vi "Teleop.vi"(10 "Match Info":T2={"Autonomous Elapsed Seconds"=0.0, "TeleOp Elapsed Seconds"=0.0, "Disabled Elapsed Seconds"=0.0, "Visited Autonomous"=FALSE, "Visited TeleOp"=FALSE, "Visited Disabled"=FALSE, "Autonomous Settings"={"Autonomous Style"=enum."Independent", "VI Refnum"=refnum}}, 11 "Call Context":T3) -> ()   [LabVIEW 2015]
doc: "This VI is called for each TeleOp packet received from the DS where the robot is not disabled. It is often used to read from the joysticks and update I/O or to update setpoints for timed control loops. It should complete and return within 20 milliseconds or it may miss DS packets."
uses:
  <vilib>/Rock Robotics/WPI/DriverStation/WPI_DriverStationDerivedRobotMode.ctl
  <vilib>/Rock Robotics/WPI/DriverStation/WPI_DriverStationMatch Info.ctl
  <vilib>/Rock Robotics/WPI/CAN/TalonSRX/WPI_CANTalonSRX_BrakeOverride.ctl
  <vilib>/Rock Robotics/WPI/CAN/TalonSRX/WPI_CANTalonSRX_APIControlMode.ctl
  <vilib>/Rock Robotics/WPI/Utilities/WPI_GetSetVariantRefNum.vi
  <vilib>/Rock Robotics/Network Tables/SD Write Number.vi
  <vilib>/Rock Robotics/Network Tables/NT Write Number.vi
  <vilib>/Rock Robotics/Network Tables/SD Write Boolean.vi
  <vilib>/Rock Robotics/WPI/Solenoid/Deprecated/WPI_SolenoidSetBool.vi
  Robot Global Data.vi
  <vilib>/addons/control/pid/pid.llb/PID (DBL).vi
  navX Library v2/navX Library v2.lvlib
  <vilib>/addons/control/pid/NI_PID_pid.lvlib
panel:
  in  "RPM":dbl
  in  "Aiming Gains":T1={"proportional gain (Kc)"=1.0, "integral time (Ti, min)"=0.01, "derivative time (Td, min)"=0.0} {"derivative time (Td, min)" format="%.3f"; "integral time (Ti, min)" format="%.3f"; "proportional gain (Kc)" format="%.3f"}
  out "Displacement X":dbl
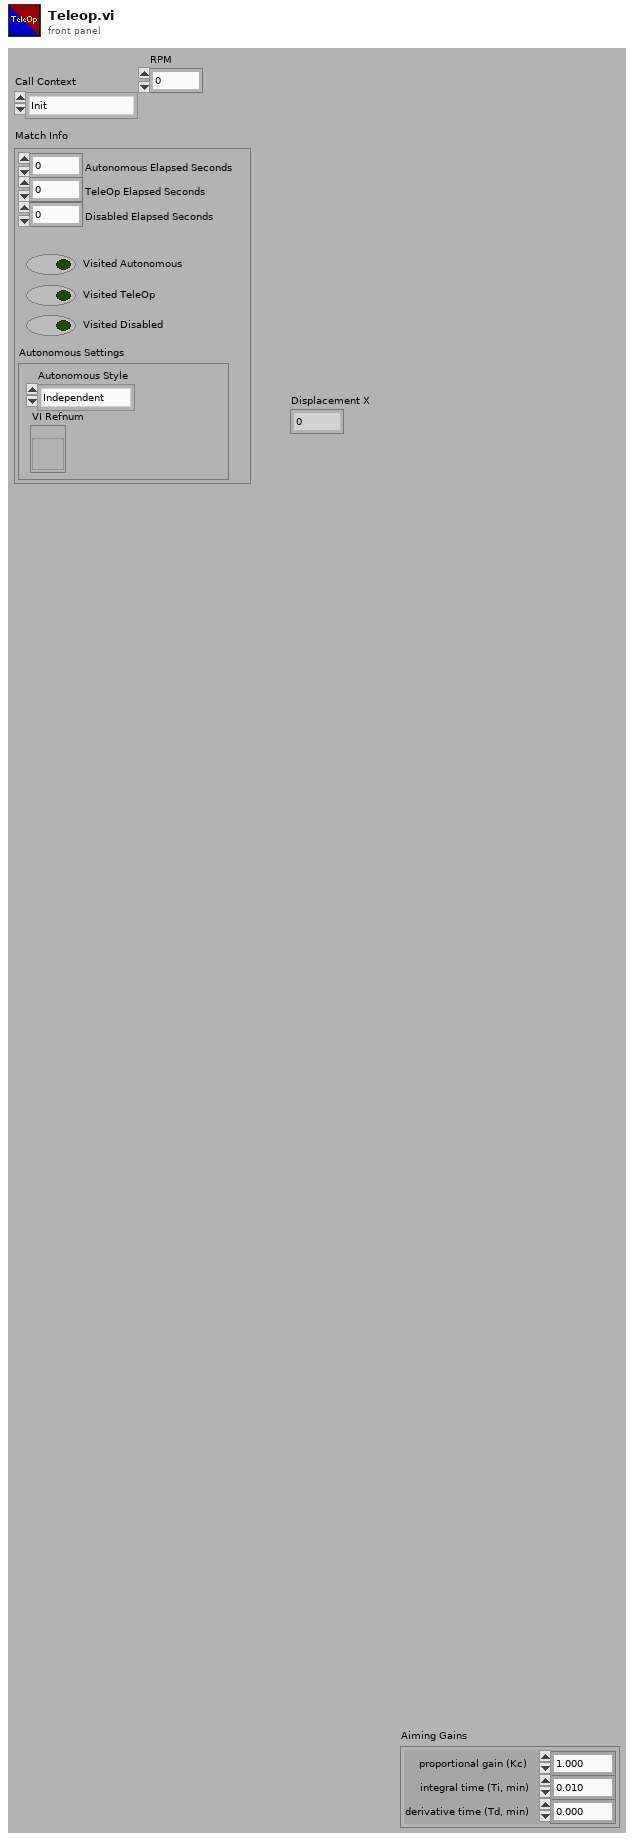
[diagram p1: front panel]
types:
  T1 = cluster{"proportional gain (Kc)":dbl, "integral time (Ti, min)":dbl, "derivative time (Td, min)":dbl}
  T2 = typedef "WPI_DriverStationMatch Info.ctl" = cluster{"Autonomous Elapsed Seconds":dbl, "TeleOp Elapsed Seconds":dbl, "Disabled Elapsed Seconds":dbl, "Visited Autonomous":bool, "Visited TeleOp":bool, "Visited Disabled":bool, "Autonomous Settings":cluster{"Autonomous Style":enum16{"Iterative", "Independent"}, "VI Refnum":refnum<vi>}}
  T3 = typedef "WPI_DriverStationDerivedRobotMode.ctl" = enum16{"Init", "Execute", "Stop"}
  T4 = typedef "WPI_CANTalonSRX_BrakeOverride.ctl" = enum8{"No Override", "Override to Coast", "Override to Brake"}
  T5 = typedef "WPI_MotorControlDeviceRef.ctl" = cluster{"DeviceStatus":errorcluster, "Type":T6, "PWM":cluster{"PWM Channel":T7, "DeadBand":T8}, "CAN":cluster{"Device Number":u8, "Control Mode":T9, "Semaphore":T10, "Max Vout":dbl, "TalonSRX Control Mode":T11}, "Invert":bool}
  T6 = typedef "WPI_MotorControlType.ctl" = enum16{"PWM", "CAN", "CANTalonSRX"}
  T7 = typedef "FPGA_DIOPWMChannel.ctl" = enum8{"PWM 0", "PWM 1", "PWM 2", "PWM 3", "PWM 4", "PWM 5", "PWM 6", "PWM 7", "PWM 8", "PWM 9", "PWM MXP 0", "PWM MXP 1", "PWM MXP 2", "PWM MXP 3", "PWM MXP 4", "PWM MXP 5", "PWM MXP 6", "PWM MXP 7", "PWM MXP 8", "PWM MXP 9", "Invalid"}
  T8 = typedef "WPI_PWMDeadband.ctl" = cluster{"Name":string, "maxPositivePwm":i32, "minPositivePwm":i32, "centerPwm":i32, "maxNegativePwm":i32, "minNegativePwm":i32, "angularRange":u16}
  T9 = typedef "WPI_CANJaguar_ControlMode.ctl" = enum8{"Percent VBus", "Current", "Speed", "Position", "Voltage"}
  T10 = typedef "Semaphore RefNum" = refnum<k1>
  T11 = typedef "WPI_CANTalonSRX_APIControlMode.ctl" = enum8{"Percent VBus", "Speed", "Position", "Slave", "Unchanged / Invalid", "Voltage Compensation", "Current", "Motion Profile"}
  T12 = typedef "navX Library v2.lvlib/Z900_navX_DeviceTypeDef.ctl" = cluster{"Interface":cluster{"Protocol":T13, "Update Rate (4Hz-60Hz)":u8, "navX Open TypeDef":variant}, "Notify Packet":refnum<notifier>, "Loop VI Refnum":refnum<vi>, "Ready to Close Occurrence Refnum":refnum<k4>}
  T13 = typedef "navX Library v2.lvlib/Z900_navX_ProtocolTypeDef.ctl" = enum16{"SERIAL", "I2C", "SPI"}
  T14 = cluster{"Yaw":dbl, "Roll":dbl, "Pitch":dbl, "Heading":dbl, "Fused Heading":dbl}
  T15 = cluster{"LinearAcceleration X":dbl, "LinearAcceleration Y":dbl, "LinearAcceleration Z":dbl}
  T16 = typedef "WPI_JoystickDevRef.ctl" = cluster{"Device":T17}
  T17 = typedef "WPI_JoystickDeviceEnum.ctl" = enum16{"USB 0", "USB 1", "USB 2", "USB 3", "USB 4", "USB 5"}
  T18 = cluster{"Velocity X":dbl, "Velocity Y":dbl, "Velocity Z":dbl, "Displacement X":dbl, "Displacement Y":dbl, "Displacement Z":dbl}
  T19 = cluster{"Axes[0]":dbl, "Axes[1]":dbl, "Axes[2]":dbl, "Axes[3]":dbl, "Axes[4]":dbl, "Axes[5]":dbl, "Axes[6]":dbl, "Axes[7]":dbl, "Axes[8]":dbl}
  T20 = cluster{"Buttons[0]":bool, "Buttons[1]":bool, "Buttons[2]":bool, "Buttons[3]":bool, "Buttons[4]":bool, "Buttons[5]":bool, "Buttons[6]":bool, "Buttons[7]":bool, "Buttons[8]":bool}
  T21 = typedef "WPI_CANTalonSRX_GlobalStatus.ctl" = cluster{"Applied Throttle":dbl, "Module Enabled":bool, "CAN Error":errorcluster, "Closed Loop Error":dbl, "Forward Limit Switch Closed":bool, "Reverse Limit Switch Closed":bool, "Sensor Position":dbl, "Sensor Velocity":dbl, "Current":dbl, "Sticky Fault - Over Temp":bool, "Sticky Fault - Under Voltage":bool, "Sticky Fault - Forward Limit":bool, "Sticky Fault - Reverse Limit":bool, "Sticky Fault - Forward Soft Limit":bool, "Sticky Fault - Reverse Soft Limit":bool, "Brake is Enabled":bool, "Encoder Position":dbl, "Encoder Velocity":dbl, "Encoder Index Count":dbl, "Encoder A Pin State":bool, "Encoder B Pin State":bool, "Encoder Index Pin State":bool, "Analog In":dbl, "Analog In Velocity":dbl, "Temperature (C)":dbl, "Battery Voltage":dbl, "Control 5 Is Supported":bool, "Current Profile Slot Select":dbl, "Pos Div 8":bool, "Vel Div 4":bool, "Pulse Width Position":i32, "Pulse Width Velocity":i32, "Pulse Width Rise To Rise (us)":i32, "Pulse Width Rise To Fall (us)":i32, "Mot Prof Active Is Under Run":bool, "Mot Prof Active Has Under Run":bool, "Mot Prof Active Is Last":bool, "Mot Prof Active Velocity Only":bool, "Mot Prof Active Is Valid":bool, "Mot Prof Buffer Is Full":bool, "Mot Prof Active Profile Slot Select":i32, "Mot Prof NextID":i32, "Mot Prof Count":i32, "Mot Prof Active Velocity":dbl, "Mot Prof Active Position":dbl, "Mot Prof Output Enable":i32}
  T22 = typedef "WPI_SolenoidDevRef.ctl" = cluster{"DevStatus":errorcluster, "Pneumatics Control Module":u8, "Forward Solenoid Channel":T23, "Reverse Solenoid Channel":T23}
  T23 = typedef "WPI_SolenoidChannel.ctl" = enum8{"Solenoid 0", "Solenoid 1", "Solenoid 2", "Solenoid 3", "Solenoid 4", "Solenoid 5", "Solenoid 6", "Solenoid 7", "Invalid"}
  T24 = typedef "WPI_RobotDriveDevRef.ctl" = cluster{"DevStatus":errorcluster, "Motors[]":T5[], "Square Inputs":bool, "Max Output":dbl}
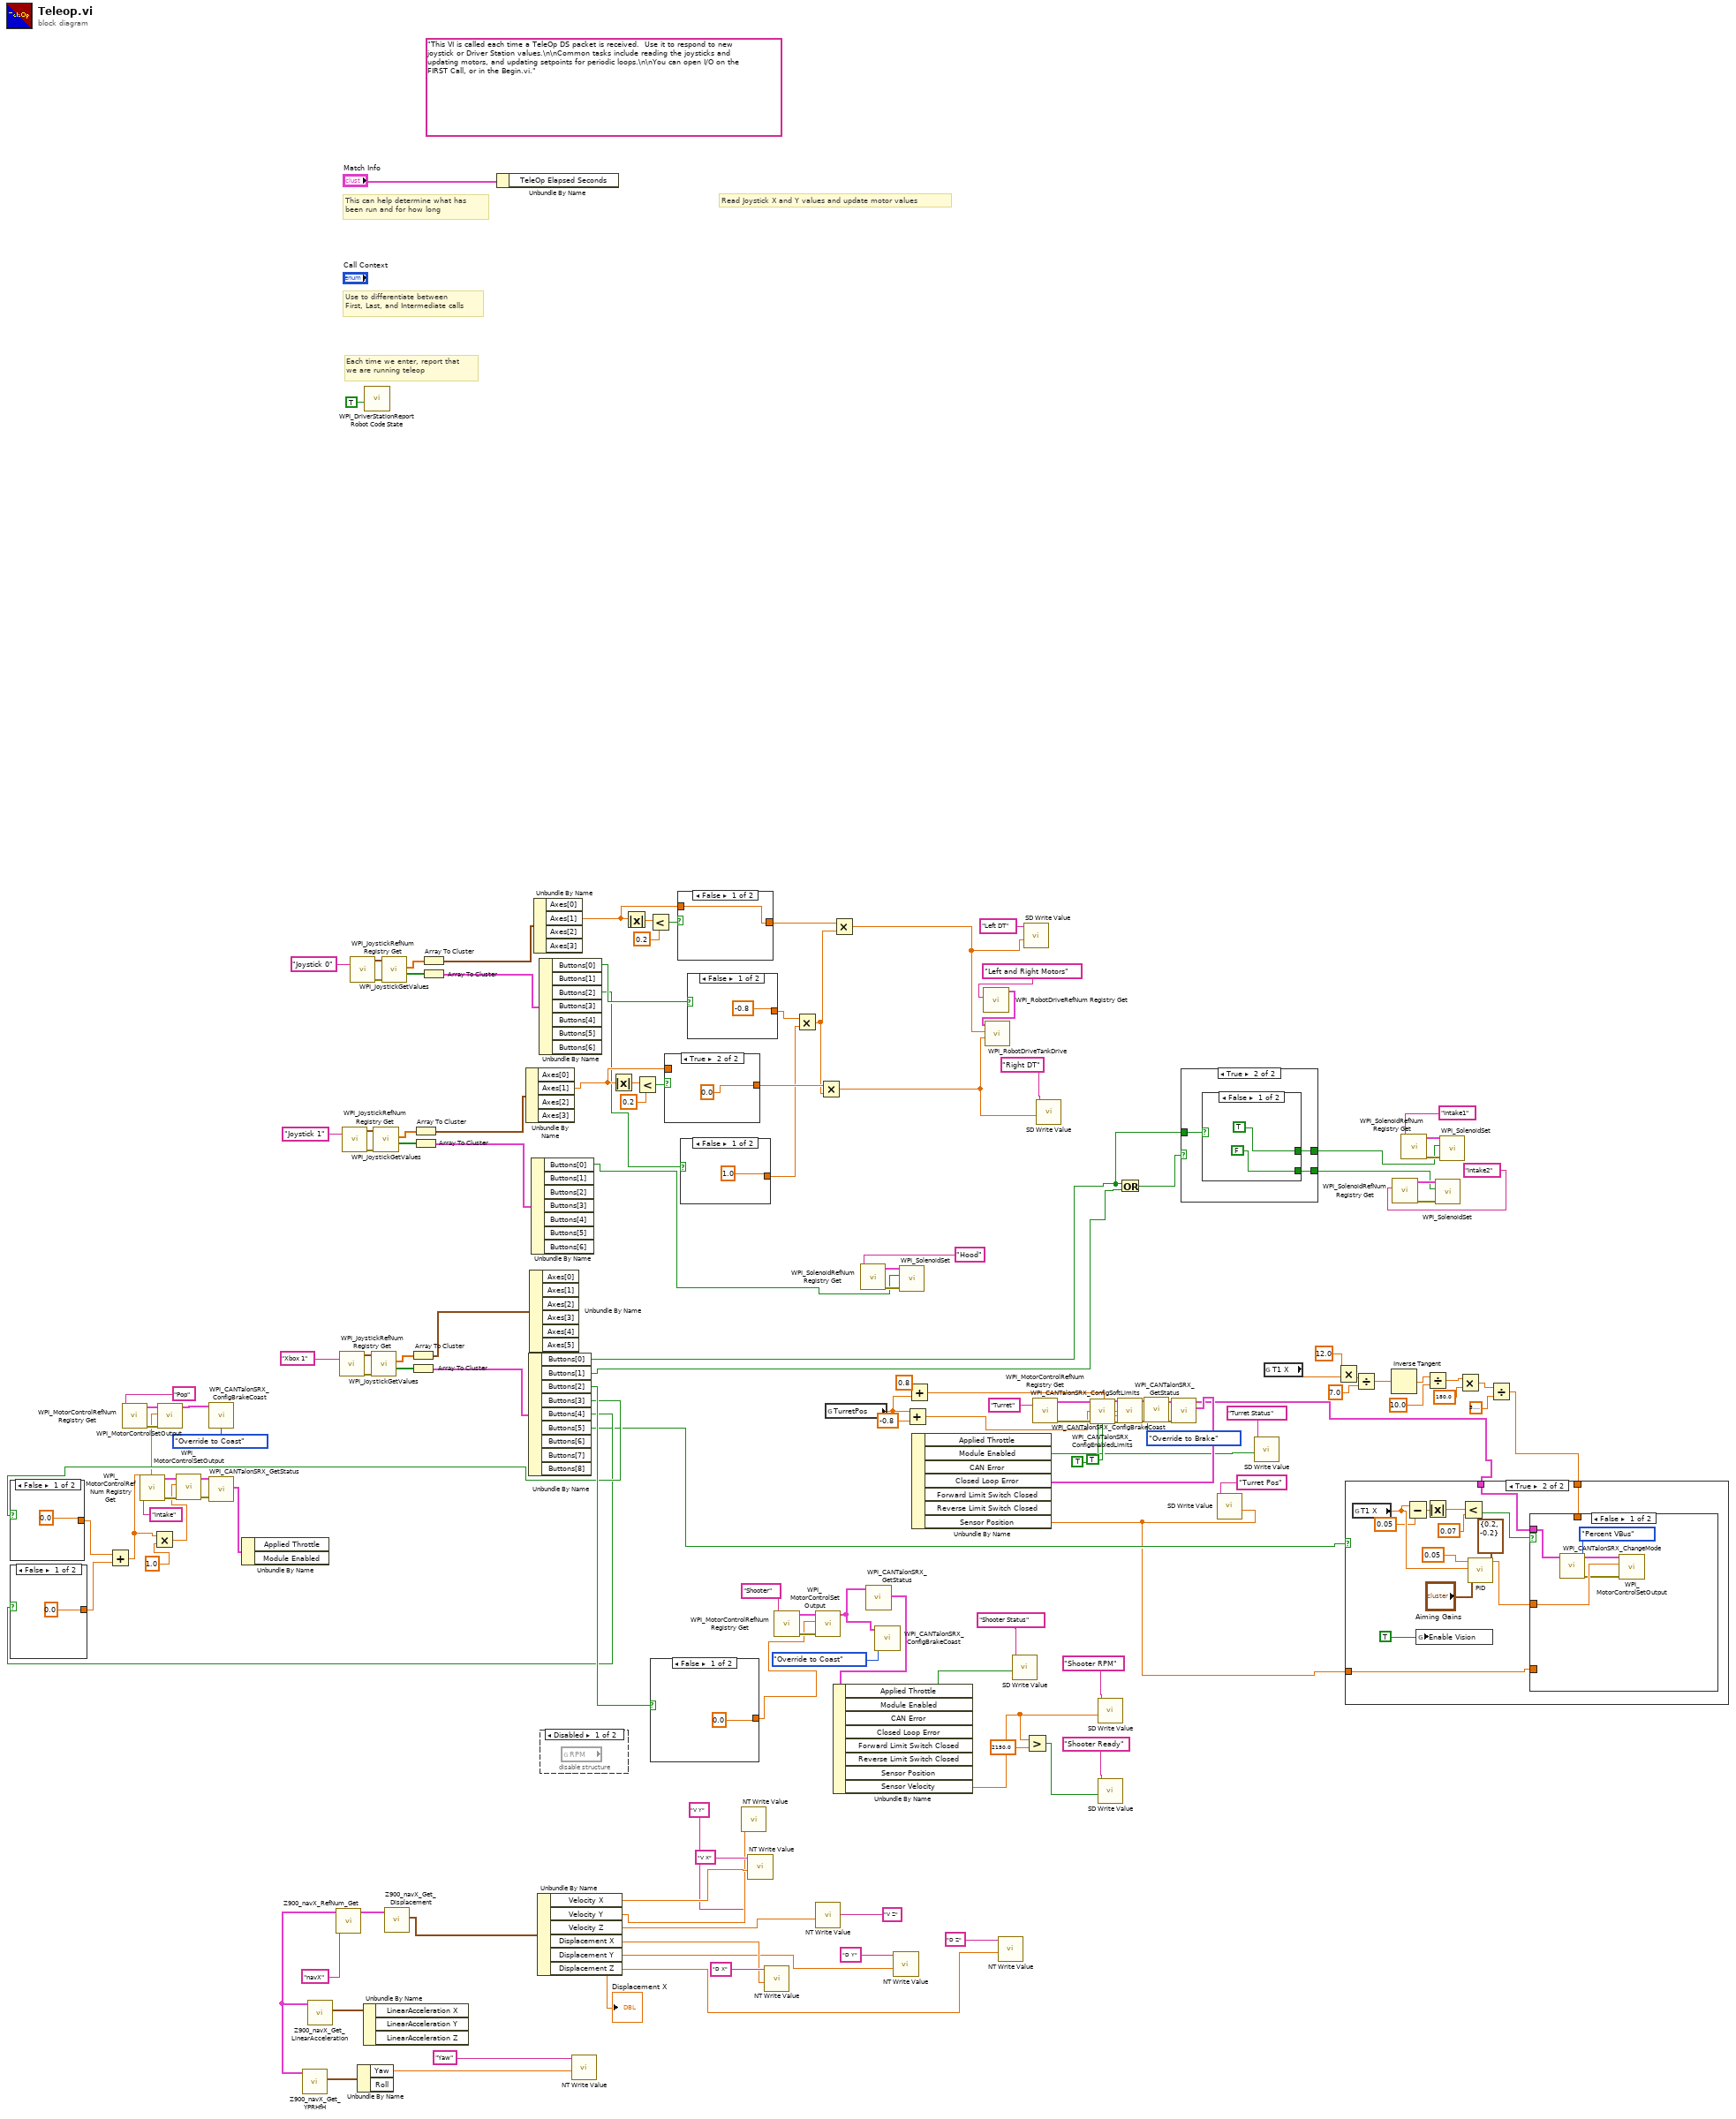
[diagram p0: block diagram]
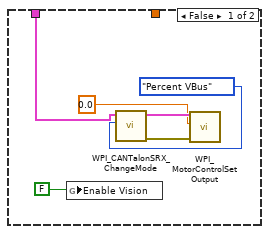
[diagram p2: hidden frame]
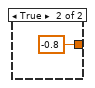
[diagram p5: hidden frame]
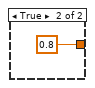
[diagram p6: hidden frame]
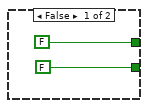
[diagram p7: hidden frame]
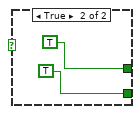
[diagram p8: hidden frame]
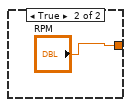
[diagram p9: hidden frame]
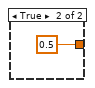
[diagram p10: hidden frame]
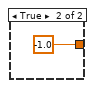
[diagram p11: hidden frame]
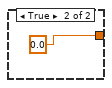
[diagram p13: hidden frame]
diagram:
  (unwired) "This VI is called each time a TeleOp DS packet is received.  Use it to respond to new joystick or Driver Station values.\n\nCommon tasks include reading the joysticks and updating motors, and updating setpoints for periodic loops.\n\nYou can open I/O on the FIRST Call, or in the Begin.vi."
  # "Each time we enter, report that\nwe are running teleop"
  # "Use to differentiate between\nFirst, Last, and Intermediate calls"
  # "This can help determine what has\nbeen run and for how long"
  # "Read Joystick X and Y values and update motor values"
  n1 = call <vilib>:"WPI_MotorControlRefNum Registry Get.vi"("refnum name"="Pop") -> ("error out"=w21:errorcluster, "MotorControlDevRef"=w22:T5)  [unwired: 9 in]
  n2 = call <vilib>:"WPI_MotorControlRefNum Registry Get.vi"("refnum name"="Intake") -> ("error out"=w23:errorcluster, "MotorControlDevRef"=w24:T5)  [unwired: 9 in]
  n3 = call "Z900_navX_RefNum_Get.vi"("refnum name"="navX") -> ("navX Device"=w102:T12)  [unwired: 9 in, 1 out]
  n4 = call "Z900_navX_Get_YPRHfH.vi"("navX Device"=w102) -> ("YRPHfH"=w101:T14)  [unwired: 7 in, 3 out]
  n5 = call "Z900_navX_Get_LinearAcceleration.vi"("navX Device"=w102) -> ("Linear Acceleration"=w109:T15)  [unwired: 7 in, 3 out]
  n6 = call <vilib>:"WPI_JoystickRefNum Registry Get.vi"("refnum name"="Xbox 1") -> ("error out"=w91:errorcluster, "JoystickDevRef"=w90:T16)  [unwired: 9 in]
  n7 = call <vilib>:"WPI_JoystickRefNum Registry Get.vi"("refnum name"="Joystick 1") -> ("error out"=w137:errorcluster, "JoystickDevRef"=w136:T16)  [unwired: 9 in]
  n8 = call <vilib>:"WPI_JoystickRefNum Registry Get.vi"("refnum name"="Joystick 0") -> ("error out"=w144:errorcluster, "JoystickDevRef"=w143:T16)  [unwired: 9 in]
  n9 = Unbundle By Name(w101) -> ("Yaw"=w99:dbl)  [unwired: 1 out]
  n10 = Unbundle By Name(w109) -> ()  [unwired: 3 out]
  n11 = call <vilib>:"WPI_DriverStationReport Robot Code State.vi"("TeleOp"=TRUE ("Autonomous")) -> ()  [unwired: 10 in, 1 out]
  n12 = call <vilib>:"WPI_JoystickGetValues.vi"("error in (no error)"=w91, "JoystickDevRef"=w90) -> ("Buttons"=w88:bool[], "Axes"=w89:dbl[])  [unwired: 5 in, 3 out]
  n13 = call <vilib>:"WPI_JoystickGetValues.vi"("error in (no error)"=w137, "JoystickDevRef"=w136) -> ("Buttons"=w134:bool[], "Axes"=w135:dbl[])  [unwired: 5 in, 3 out]
  n14 = call <vilib>:"WPI_JoystickGetValues.vi"("error in (no error)"=w144, "JoystickDevRef"=w143) -> ("Buttons"=w141:bool[], "Axes"=w142:dbl[])  [unwired: 5 in, 3 out]
  n15 = call "Z900_navX_Get_Displacement.vi"("navX Device"=w102) -> ("Displacement"=w117:T18)  [unwired: 7 in, 3 out]
  n16 = Array To Cluster(array=w89) -> (cluster=w87:T19)
  n17 = Array To Cluster(array=w88) -> (cluster=w86:T20)
  n18 = Array To Cluster(array=w135) -> (cluster=w133:T19)
  n19 = Array To Cluster(array=w134) -> (cluster=w132:T20)
  n20 = Array To Cluster(array=w142) -> (cluster=w140:T19)
  n21 = Array To Cluster(array=w141) -> (cluster=w139:T20)
  n22 = Unbundle By Name("Match Info") -> ()  [unwired: 1 out]
  n23 = Unbundle By Name(w133) -> ("Axes[1]"=w122:dbl)  [unwired: 3 out]
  n24 = Unbundle By Name(w86) -> ("Buttons[0]"=w33:bool, "Buttons[1]"=w37:bool, "Buttons[2]"=w59:bool, "Buttons[3]"=w15:bool, "Buttons[4]"=w14:bool, "Buttons[5]"=w9:bool)  [unwired: 3 out]
  n25 = case shown="False" w15 {
    tunnel: [0.0 0.8] -> w17
    frame False {
    }
    frame True {
    }
  }
  n26 = case shown="False" w14 {
    tunnel: [0.0 -0.8] -> w16
    frame False {
    }
    frame True {
    }
  }
  n27 = Add(x=w17, y=w16) -> (x+y=w11:dbl)
  n28 = Multiply(x=w11, y=1.0) -> (x*y=w10:dbl)
  n29 = call <vilib>:"WPI_MotorControlSetOutput.vi"("error in (no error)"=w21, "Output"=w11, "MotorControlDevRef"=w22) -> ("MotorControlDevRef"=w27:T5)  [unwired: 6 in, 2 out]
  n30 = call <vilib>:"WPI_MotorControlSetOutput.vi"("error in (no error)"=w23, "Output"=w10, "MotorControlDevRef"=w24) -> ("error out"=w19:errorcluster, "MotorControlDevRef"=w20:T5)  [unwired: 6 in, 1 out]
  n31 = call <vilib>:"WPI_CANTalonSRX_ConfigBrakeCoast.vi"("Brake / Coast Mode"=WPI_CANTalonSRX_BrakeOverride."Override to Coast", "CAN Talon SRX Ref"=w27) -> ()  [unwired: 8 in, 2 out]
  n32 = call <vilib>:"WPI_CANTalonSRX_GetStatus.vi"("error in (no error)"=w19, "CAN Talon SRX Ref"=w20) -> ("Talon SRX Status"=w18:T21)  [unwired: 7 in, 2 out]
  n33 = Unbundle By Name(w18) -> ()  [unwired: 2 out]
  n34 = Unbundle By Name(w87) -> ()  [unwired: 6 out]
  n35 = Unbundle By Name(w132) -> ("Buttons[0]"=w29:bool)  [unwired: 6 out]
  n36 = Unbundle By Name(w140) -> ("Axes[1]"=w127:dbl)  [unwired: 3 out]
  n37 = Unbundle By Name(w117) -> ("Velocity X"=w115:dbl, "Velocity Y"=w113:dbl, "Velocity Z"=w110:dbl, "Displacement X"=w105:dbl, "Displacement Y"=w104:dbl, "Displacement Z"=w103:dbl)
  "Displacement X" <- w105
  n38 = Unbundle By Name(w139) -> ("Buttons[0]"=w96:bool, "Buttons[2]"=w60:bool)  [unwired: 5 out]
  n39 = disable-structure shown="Disabled" {
    frame Disabled {
      n40 = global read "Robot Global Data.vi" "RPM"() -> ()  [unwired: 1 out]
    }
    frame Enabled {
    }
  }
  n41 = call-poly <vilib>:"NT Write Value.vi"("Numeric"=w99, "Name"="Yaw") -> ()  [unwired: 9 in, 1 out]
  n42 = Absolute Value(x=w122) -> (abs(x)=w126:dbl)
  n43 = Absolute Value(x=w127) -> (abs(x)=w131:dbl)
  n44 = Less?(x=w126, y=0.2) -> (x < y?=w124:bool)
  n45 = Less?(x=w131, y=0.2) -> (x < y?=w129:bool)
  n46 = case shown="False" w59 {
    tunnel: [0.0 "RPM"] -> w58
    frame False {
    }
    frame True {
    }
  }
  n47 = case shown="True" w124 {
    tunnel: [w154 0.0] -> w123
    tunnel: w122 -> [w154 _]
    frame False {
    }
    frame True {
    }
  }
  n48 = case shown="False" w129 {
    tunnel: [w156 0.0] -> w128
    tunnel: w127 -> [w156 _]
    frame False {
    }
    frame True {
    }
  }
  n49 = case shown="False" w60 {
    tunnel: [1.0 0.5] -> w94
    frame False {
    }
    frame True {
    }
  }
  n50 = case shown="False" w96 {
    tunnel: [-0.8 -1.0] -> w95
    frame False {
    }
    frame True {
    }
  }
  n51 = call-poly <vilib>:"NT Write Value.vi"("Numeric"=w113, "Name"="V Y") -> ()  [unwired: 9 in, 1 out]
  n52 = call-poly <vilib>:"NT Write Value.vi"("Numeric"=w115, "Name"="V X") -> ()  [unwired: 9 in, 1 out]
  n53 = call-poly <vilib>:"NT Write Value.vi"("Numeric"=w105, "Name"="D X") -> ()  [unwired: 9 in, 1 out]
  n54 = call <vilib>:"WPI_MotorControlRefNum Registry Get.vi"("refnum name"="Shooter") -> ("error out"=w72:errorcluster, "MotorControlDevRef"=w71:T5)  [unwired: 9 in]
  n55 = Multiply(x=w95, y=w94) -> (x*y=w93:dbl)
  n56 = call <vilib>:"WPI_MotorControlSetOutput.vi"("error in (no error)"=w72, "Output"=w58, "MotorControlDevRef"=w71) -> ("MotorControlDevRef"=w69:T5)  [unwired: 6 in, 2 out]
  n57 = call-poly <vilib>:"NT Write Value.vi"("Numeric"=w110, "Name"="V Z") -> ()  [unwired: 9 in, 1 out]
  n58 = Multiply(x=w123, y=w93) -> (x*y=w97:dbl)
  n59 = global read "Robot Global Data.vi" "TurretPos"() -> (w5:dbl)
  n60 = Multiply(x=w128, y=w93) -> (x*y=w98:dbl)
  n61 = call <vilib>:"WPI_SolenoidRefNum Registry Get.vi"("refnum name"="Hood") -> ("error out"=w32:errorcluster, "SolenoidDevRef"=w31:T22)  [unwired: 9 in]
  n62 = call <vilib>:"WPI_CANTalonSRX_GetStatus.vi"("CAN Talon SRX Ref"=w69) -> ("Talon SRX Status"=w13:T21)  [unwired: 8 in, 2 out]
  n63 = Unbundle By Name(w13) -> ("Module Enabled"=w66:bool, "Sensor Velocity"=w63:dbl)  [unwired: 6 out]
  n64 = call <vilib>:"WPI_CANTalonSRX_ConfigBrakeCoast.vi"("Brake / Coast Mode"=WPI_CANTalonSRX_BrakeOverride."Override to Coast", "CAN Talon SRX Ref"=w69) -> ()  [unwired: 8 in, 2 out]
  n65 = call-poly <vilib>:"NT Write Value.vi"("Numeric"=w104, "Name"="D Y") -> ()  [unwired: 9 in, 1 out]
  n66 = call-poly <vilib>:"WPI_SolenoidSet.vi"("error in (no error)"=w32, "Value"=w29, "SolenoidDevRef"=w31) -> ()  [unwired: 7 in, 2 out]
  n67 = Add(x=w5, y=-0.8) -> (x+y=w2:dbl)
  n68 = Add(x=0.8, y=w5) -> (x+y=w1:dbl)
  n69 = call <vilib>:"WPI_RobotDriveRefNum Registry Get.vi"("refnum name"="Left and Right Motors") -> ("RobotDriveDevRef"=w121:T24)  [unwired: 9 in, 1 out]
  n70 = call <vilib>:"WPI_RobotDriveTankDrive.vi"("Right axis value"=w97, "Left axis value"=w98, "RobotDriveDevRef"=w121) -> ()  [unwired: 6 in, 3 out]
  n71 = call-poly <vilib>:"NT Write Value.vi"("Numeric"=w103, "Name"="D Z") -> ()  [unwired: 9 in, 1 out]
  n72 = call-poly <vilib>:"SD Write Value.vi"("Boolean"=w66, "Name"="Shooter Status") -> ()  [unwired: 8 in, 2 out]
  n73 = call-poly <vilib>:"SD Write Value.vi"("Numeric"=w98, "Name"="Left DT") -> ()  [unwired: 8 in, 2 out]
  n74 = Greater?(x=w63, y=2150.0) -> (0:w61:bool)
  n75 = call <vilib>:"WPI_MotorControlRefNum Registry Get.vi"("refnum name"="Turret") -> ("error out"=w46:errorcluster, "MotorControlDevRef"=w45:T5)  [unwired: 9 in]
  n76 = call-poly <vilib>:"SD Write Value.vi"("Numeric"=w97, "Name"="Right DT") -> ()  [unwired: 8 in, 2 out]
  n77 = call <vilib>:"WPI_CANTalonSRX_ConfigEnabledLimits.vi"("CAN Talon SRX Ref"=w45, "error in (no error)"=w46, "Forward Soft Limit Enable"=TRUE, "Reverse Soft Limit Enable"=TRUE) -> ("CAN Talon SRX Ref"=w44:T5, "error out"=w82:errorcluster)  [unwired: 10 in]
  n78 = call-poly <vilib>:"SD Write Value.vi"("Numeric"=w63, "Name"="Shooter RPM") -> ()  [unwired: 8 in, 2 out]
  n79 = call-poly <vilib>:"SD Write Value.vi"("Boolean"=w61, "Name"="Shooter Ready") -> ()  [unwired: 8 in, 2 out]
  n80 = call <vilib>:"WPI_CANTalonSRX_ConfigSoftLimits.vi"("CAN Talon SRX Ref"=w44, "Forward Limit Position"=w2, "Reverse Limit Position"=w1, "error in (no error)"=w82) -> ("CAN Talon SRX Ref"=w80:T5, "error out"=w81:errorcluster)  [unwired: 10 in]
  n81 = Or(x=w33, y=w37) -> (x .or. y?=w36:bool)
  n82 = call <vilib>:"WPI_CANTalonSRX_ConfigBrakeCoast.vi"("error in (no error)"=w81, "Brake / Coast Mode"=WPI_CANTalonSRX_BrakeOverride."Override to Brake", "CAN Talon SRX Ref"=w80) -> ("error out"=w78:errorcluster, "CAN Talon SRX Ref"=w77:T5)  [unwired: 7 in]
  n83 = call <vilib>:"WPI_CANTalonSRX_GetStatus.vi"("error in (no error)"=w78, "CAN Talon SRX Ref"=w77) -> ("Talon SRX Status"=w76:T21, "CAN Talon SRX Ref"=w7:T5)  [unwired: 7 in, 1 out]
  n84 = Unbundle By Name(w76) -> ("Module Enabled"=w74:bool, "Sensor Position"=w8:dbl)  [unwired: 5 out]
  n85 = case shown="True" w36 {
    tunnel: [FALSE w165] -> w35
    tunnel: [FALSE w164] -> w34
    tunnel: w33 -> [_ w166]
    frame False {
    }
    frame True {
      n86 = case shown="False" w166 {
        tunnel: [TRUE TRUE] -> w165
        tunnel: [FALSE TRUE] -> w164
        frame False {
        }
        frame True {
        }
      }
    }
  }
  n87 = call-poly <vilib>:"SD Write Value.vi"("Numeric"=w8, "Name"="Turret Pos") -> ()  [unwired: 8 in, 2 out]
  n88 = call-poly <vilib>:"SD Write Value.vi"("Boolean"=w74, "Name"="Turret Status") -> ()  [unwired: 8 in, 2 out]
  n89 = global read "Robot Global Data.vi" "T1 X"() -> (w55:dbl)
  n90 = Multiply(x=w55, y=12.0) -> (x*y=w53:dbl)
  n91 = Divide(x=w53, y=7.0) -> (x/y=w57:dbl)
  n92 = Inverse Tangent(1:w57) -> (0:w52:dbl)
  n93 = call <vilib>:"WPI_SolenoidRefNum Registry Get.vi"("refnum name"="Intake2") -> ("error out"=w39:errorcluster, "SolenoidDevRef"=w40:T22)  [unwired: 9 in]
  n94 = call <vilib>:"WPI_SolenoidRefNum Registry Get.vi"("refnum name"="Intake1") -> ("error out"=w41:errorcluster, "SolenoidDevRef"=w42:T22)  [unwired: 9 in]
  n95 = Divide(x=w52, y=10.0) -> (x/y=w50:dbl)
  n96 = call-poly <vilib>:"WPI_SolenoidSet.vi"("error in (no error)"=w39, "Value"=w34, "SolenoidDevRef"=w40) -> ()  [unwired: 7 in, 2 out]
  n97 = call-poly <vilib>:"WPI_SolenoidSet.vi"("error in (no error)"=w41, "Value"=w35, "SolenoidDevRef"=w42) -> ()  [unwired: 7 in, 2 out]
  n98 = Multiply(x=w50, y=180.0) -> (x*y=w48:dbl)
  n99 = Divide(x=w48, y=3.141592653589793) -> (x/y=w6:dbl)
  n100 = case shown="True" w9 {
    tunnel: w7 -> [w173 w183]
    tunnel: w8 -> [_ w182]
    tunnel: w6 -> [_ w181]
    frame False {
      n101 = global write "Robot Global Data.vi" "Enable Vision"(FALSE) -> ()
      n102 = call <vilib>:"WPI_CANTalonSRX_ChangeMode.vi"("Control Mode"=WPI_CANTalonSRX_APIControlMode."Percent VBus", "CAN Talon SRX Ref"=w173) -> ("error out"=w175:errorcluster, "CAN Talon SRX Ref"=w176:T5)  [unwired: 8 in]
      n103 = call <vilib>:"WPI_MotorControlSetOutput.vi"("error in (no error)"=w175, "Output"=0.0, "MotorControlDevRef"=w176) -> ()  [unwired: 6 in, 3 out]
    }
    frame True {
      n104 = global read "Robot Global Data.vi" "T1 X"() -> (w179:dbl)
      n105 = Subtract(x=w179, y=0.05) -> (x-y=w180:dbl)
      n106 = global write "Robot Global Data.vi" "Enable Vision"(TRUE) -> ()
      n107 = Absolute Value(x=w180) -> (abs(x)=w190:dbl)
      n108 = Less?(x=w190, y=0.07) -> (x < y?=w188:bool)
      n109 = call-poly <vilib>:"PID.vi"("output range"=cluster{"output high":dbl, "output low":dbl} {"output high"=0.2, "output low"=-0.2}, "PID gains"="Aiming Gains", "process variable"=w179, "setpoint"=0.05) -> ("output"=w184:dbl)  [unwired: 6 in, 1 out]
      n110 = case shown="False" w188 {
        tunnel: w184 -> [w194 _]
        tunnel: w183 -> [w191 _]
        tunnel: w182 -> [_ _]
        tunnel: w181 -> [_ _]
        frame False {
          n111 = call <vilib>:"WPI_CANTalonSRX_ChangeMode.vi"("Control Mode"=WPI_CANTalonSRX_APIControlMode."Percent VBus", "CAN Talon SRX Ref"=w191) -> ("error out"=w192:errorcluster, "CAN Talon SRX Ref"=w193:T5)  [unwired: 8 in]
          n112 = call <vilib>:"WPI_MotorControlSetOutput.vi"("error in (no error)"=w192, "Output"=w194, "MotorControlDevRef"=w193) -> ()  [unwired: 6 in, 3 out]
        }
        frame True {
        }
      }
    }
  }
